vi "get_setpoint.vi"(8 "error in (no error)":errorcluster, 11 "VISA Refnum in":refnum<visa-resource-name>) -> (0 "error out":errorcluster, 3 "VISA Refnum out":refnum<visa-resource-name>)   [LabVIEW 2018]
panel:
  out "Setpoint (C)":dbl
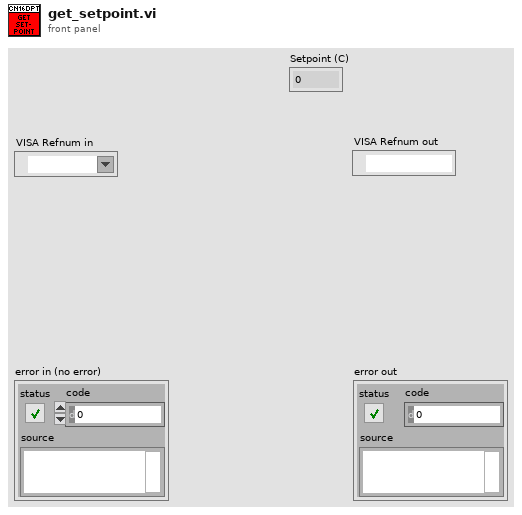
[diagram p1: front panel]
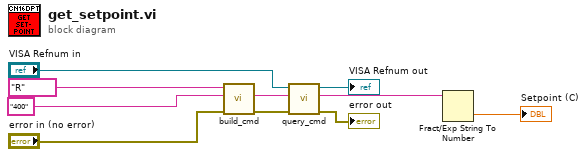
[diagram p0: block diagram]
diagram:
  n1 = call "build_cmd.vi"("error in (no error)"="error in (no error)", "Command ID"="400", "Command class"="R") -> ("error out"=w5:errorcluster, "Command"=w4:string)  [unwired: 7 in]
  n2 = call "query_cmd.vi"("error in (no error)"=w5, "Command"=w4, "VISA resource name"="VISA Refnum in") -> ("error out"=→"error out":errorcluster, "Response"=w2:string, "VISA resource name out"=→"VISA Refnum out":refnum<visa-resource-name>)  [unwired: 6 in]
  n3 = Fract/Exp String To Number(string=w2) -> (number=→"Setpoint (C)":dbl)  [unwired: 3 in, 1 out]
